vi "Init Device.vi"(7 "Layout Ref":refnum<vi>, 8 "error in (no error)":errorcluster, 10 "Chan# Array":i32[](array[numeric]), 11 "ArduinoDAC in":refnum<class "ArduinoDAC.lvclass">) -> (0 "error out":errorcluster, 3 "ArduinoDAC out":refnum<class "ArduinoDAC.lvclass">)   [LabVIEW 2013, in "ArduinoDAC.lvclass"]
doc: "Initialize the correct columns and their default appearance.\nUse the front panel to change default appearance of the device in the Add/Manage devices.\n\nOpen a specific device implementation for details."
uses:
  ArduinoDAC.lvclass
  ColumnVIs/Column/Column.lvclass
  ColumnVIs/SingleValCol/SingleValCol.lvclass
  TypeDefs/ColumnAppearCluster.ctl
panel:
  in  "Steps":T1={"Column Name"="", "Width"=30, "Bkgd"=[16448250], "Text"=[0]}
  in  "EndV":T1={"Column Name"="", "Width"=30, "Bkgd"=[16448250], "Text"=[0]}
  in  "StartV":T1={"Column Name"="", "Width"=30, "Bkgd"=[16448250], "Text"=[0]}
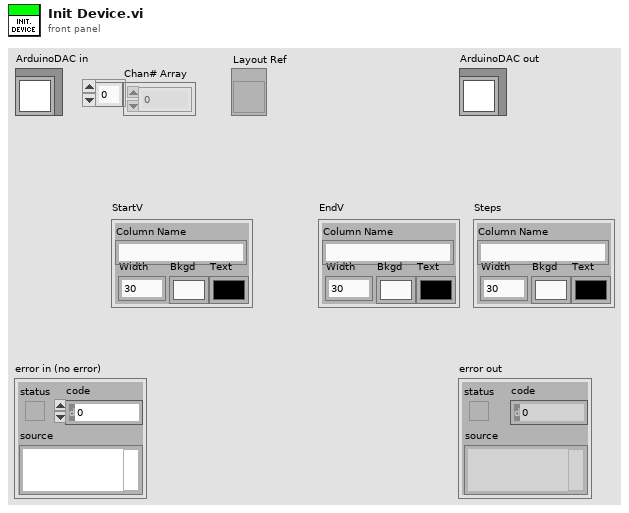
[diagram p1: front panel]
types:
  T1 = typedef "ColumnAppearCluster.ctl" = cluster{"Column Name":string, "Width":u32, "Bkgd":u32[], "Text":u32[]}
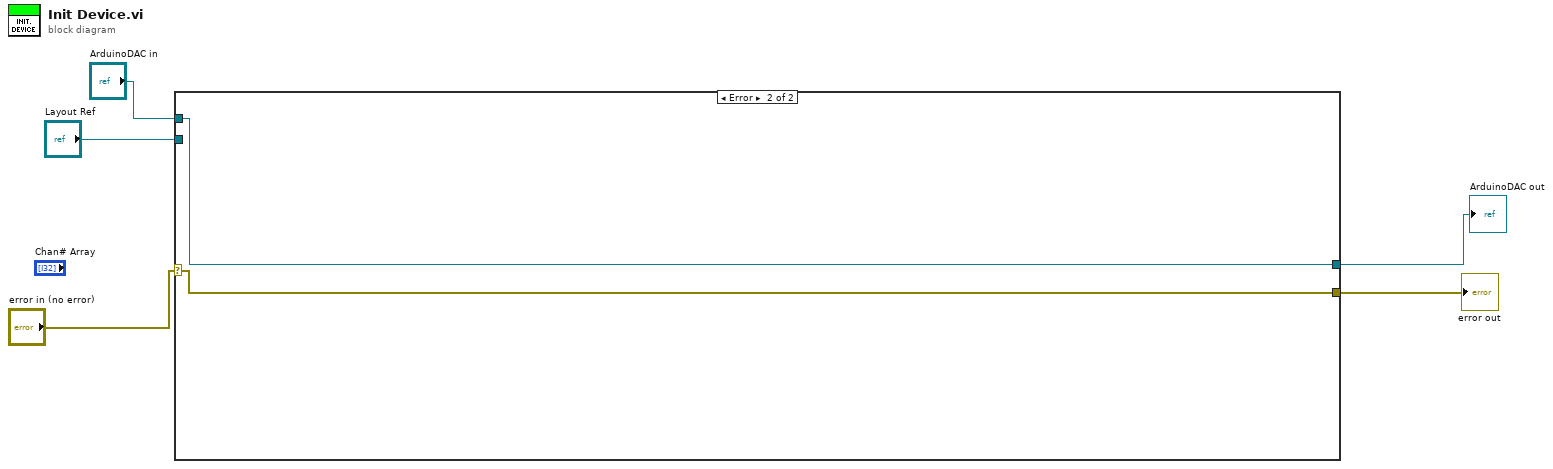
[diagram p0: block diagram]
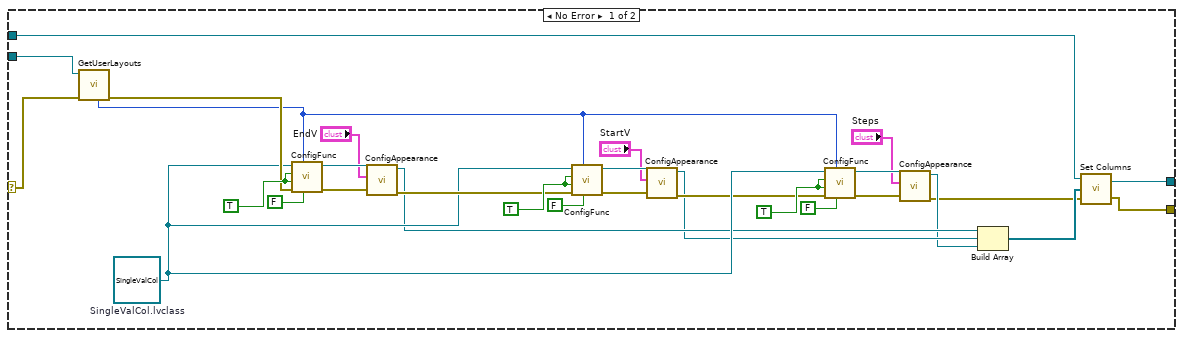
[diagram p2: hidden frame]
diagram:
  n1 = case shown="Error" "error in (no error)" {
    selector: "error in (no error)" -> [w34 w36]
    tunnel: "Layout Ref" -> [w35 _]
    tunnel: "ArduinoDAC in" -> [w9 w37]
    tunnel: [w7 w36] -> w2
    tunnel: [w6 w37] -> w1
    frame No Error {
      w23 = TRUE ("isVariable? (True)")
      w27 = TRUE ("isVariable? (True)")
      w33 = TRUE ("isVariable? (True)")
      w18 = refnum<class "SingleValCol.lvclass"> refnum  # SingleValCol.lvclass
      n2 = call "GetUserLayouts.vi"("error in (no error)"=w34, "Layout Ring Refnum"=w35) -> ("error out"=w31:errorcluster, "Num User Layouts"=w14:i32)  [unwired: 5 in, 3 out]
      n3 = call "ConfigFunc.vi"("isRampable? (True"=FALSE, "Num Layouts (ignored)"=w14, "error in (no error)"=w31, "isVariable? (True)"=w33, "Disableable? (True)"=w33, "Column in"=w18) -> ("error out"=w29:errorcluster, "Column out"=w30:refnum<class "SingleValCol.lvclass">)  [unwired: 4 in]
      n4 = call "ConfigAppearance.vi"("error in (no error)"=w29, "Column Appearance"="EndV", "Column in"=w30) -> ("error out"=w19:errorcluster, "Column out"=w13:refnum<class "SingleValCol.lvclass">)  [unwired: 7 in]
      n5 = call "ConfigFunc.vi"("isRampable? (True"=FALSE, "Num Layouts (ignored)"=w14, "error in (no error)"=w19, "isVariable? (True)"=w27, "Disableable? (True)"=w27, "Column in"=w18) -> ("error out"=w24:errorcluster, "Column out"=w25:refnum<class "SingleValCol.lvclass">)  [unwired: 4 in]
      n6 = call "ConfigAppearance.vi"("error in (no error)"=w24, "Column Appearance"="StartV", "Column in"=w25) -> ("error out"=w17:errorcluster, "Column out"=w12:refnum<class "SingleValCol.lvclass">)  [unwired: 7 in]
      n7 = call "ConfigFunc.vi"("isRampable? (True"=FALSE, "Num Layouts (ignored)"=w14, "error in (no error)"=w17, "isVariable? (True)"=w23, "Disableable? (True)"=w23, "Column in"=w18) -> ("error out"=w20:errorcluster, "Column out"=w21:refnum<class "SingleValCol.lvclass">)  [unwired: 4 in]
      n8 = call "ConfigAppearance.vi"("error in (no error)"=w20, "Column Appearance"="Steps", "Column in"=w21) -> ("error out"=w8:errorcluster, "Column out"=w11:refnum<class "SingleValCol.lvclass">)  [unwired: 7 in]
      n9 = Build Array(w13, w12, w11) -> (w10:refnum<class "SingleValCol.lvclass">[])
      n10 = call-dynamic "Set Columns.vi"("error in (no error)"=w8, "Columns"=w10, "Device in"=w9) -> ("error out"=w7:errorcluster, "Device out"=w6:refnum<class "ArduinoDAC.lvclass">)  [unwired: 1 in]
    }
    frame Error {
    }
  }
  "error out" <- w2
  "ArduinoDAC out" <- w1
